vi "defineAttributes.vi"(7 "Controls Cluster":T1(array[cluster]), 8 "error in (no error)":errorcluster, 11 "Class Reference":refnum<vi>) -> (0 "error out":errorcluster, 3 "Class Reference out":refnum<vi>)   [LabVIEW 2009, in "HGF_VisitorGenerator.lvlib"]
doc: "add attributes to visitor (controls and indicators linked to agents public interface VI conPane)"
uses:
  <vilib>/Utility/miscctls.llb/LVPositionTypeDef.ctl
  <vilib>/Utility/miscctls.llb/LVPointTypeDef.ctl
  HGF_VisitorGenerator.lvlib
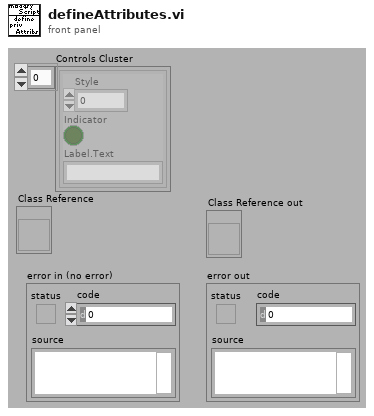
[diagram p1: front panel]
types:
  T1 = cluster{"Style":u32, "Indicator":bool, "Label.Text":string}[]
  T2 = typedef "LVPositionTypeDef.ctl" = cluster{"Left":i32, "Top":i32}
  T3 = typedef "LVPointTypeDef.ctl" = cluster{"Horizontal":i16, "Vertical":i16}
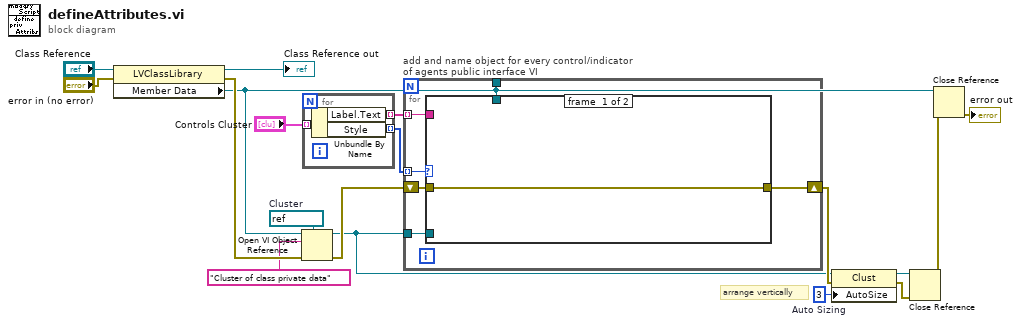
[diagram p0: block diagram]
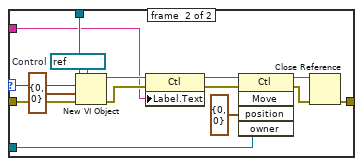
[diagram p2: hidden frame]
diagram:
  w13 = u32 3  # Auto Sizing
  w10 = refnum<vi> refnum  # Cluster
  # "arrange vertically"
  n1 = property class="LVClassLibrary"(reference="Class Reference", error in="error in (no error)") -> (reference out=→"Class Reference out":refnum<vi>, error out=w17:errorcluster, "Member Data"=w9:refnum<vi>)
  n2 = Open VI Object Reference(7:w10, 8:w17, 10:"Cluster of class private data" ("name/order"), 11:w9) -> (0:w18:errorcluster, 3:w12:refnum<vi>)
  n3 = for {
    tunnel: "Controls Cluster" -> [w21] mode=indexing
    tunnel: [w20] -> w3 mode=indexing
    tunnel: [w19] -> w2 mode=indexing
    n4 = Unbundle By Name(w21) -> ("Label.Text"=w19:string, "Style"=w20:u32)
  }
  n5 = for "add and name object for every control/indicator of agents public interface VI" {
    tunnel: w9 -> [w27]
    tunnel: w12 -> [w26]
    tunnel: w3 -> [w22] mode=indexing
    shift-right: [w25] -> w15
    shift-left: w18 -> [w24]
    tunnel: w2 -> [w23] mode=indexing
    n6 = case shown="Default" w22 {
      selector: w22 -> [_ w32]
      tunnel: w27 -> [_ w41]
      tunnel: w26 -> [_ w39]
      tunnel: [w28 w30] -> w25
      tunnel: w24 -> [w28 w38]
      tunnel: w23 -> [_ w33]
      frame #0 {
      }
      frame #1 {
        w43 = refnum<vi> refnum  # Control
        n7 = New VI Object(vi object class=w43, owner refnum=w41, style=w32, position/next to=T3 {"Horizontal"=0, "Vertical"=0} ("relative position/next to refnum"), 8:w38) -> (object refnum=w37:refnum<vi>, 0:w36:errorcluster)  [unwired: 3 in]
        n8 = property class="Ctl"(reference=w37, error in=w36, "Label.Text"=w33) -> (reference out=w34:refnum<vi>, error out=w35:errorcluster)
        n9 = invoke class="Ctl" method="Move"(reference=w34, error in=w35, "position"=T2 {"Left"=0, "Top"=0}, "owner"=w39) -> (reference out=w29:refnum<vi>, error out=w31:errorcluster)  [unwired: 1 in, 3 out]
        n10 = Close Reference(reference=w29, error in (no error)=w31) -> (error out=w30:errorcluster)
      }
    }
  }
  n11 = property class="Clust"(reference=w12, error in=w15, "AutoSize"=w13) -> (reference out=w14:refnum<vi>, error out=w16:errorcluster)
  n12 = Close Reference(reference=w14, error in (no error)=w16) -> (error out=w1:errorcluster)
  n13 = Close Reference(reference=w9, error in (no error)=w1) -> (error out=→"error out":errorcluster)
